vi "stim points to waveform.vi"(0 "stim point array":cluster{"X":u32, "Y":u32}[](array[cluster])=[{"X"=160, "Y"=192}, {"X"=107, "Y"=81}], 1 "stim power (%)":dbl(slide) scale=0.0..100.0, 2 "stim duration (in seconds)":dbl=5e-05 min=1e-05 max=0.002 step=1e-05 format="%#_6p", 3 "spot repetitions":dbl=1.0 min=1.0 step=1.0, 4 "group repetitions":dbl=1.0 min=1.0 step=1.0, 5 "pockels cell max power":dbl, 7 "stim interval (in seconds)":dbl=5e-05 min=5e-05 max=1.0 step=0.005 format="%#_6p", 9 "pre-stim settling time (in seconds)":dbl=5e-05 min=0.0 max=0.1 step=0.0001 format="%#_6p") -> (14 "x-y mirror data out":waveform(dbl)[](array[waveform]), 15 "pockels and piezo data out":waveform(dbl)[](array[waveform]), 16 "repetitions":dbl)   [LabVIEW 2012]
doc: "SciScan 1.2 160622"
panel:
  out "Waveform Graph 2":dbl[](graph)
  out "error out":errorcluster
  out "Waveform Graph":dbl[](graph)
  out "xyvoltagefor2frames":dbl[][][](array[numeric])
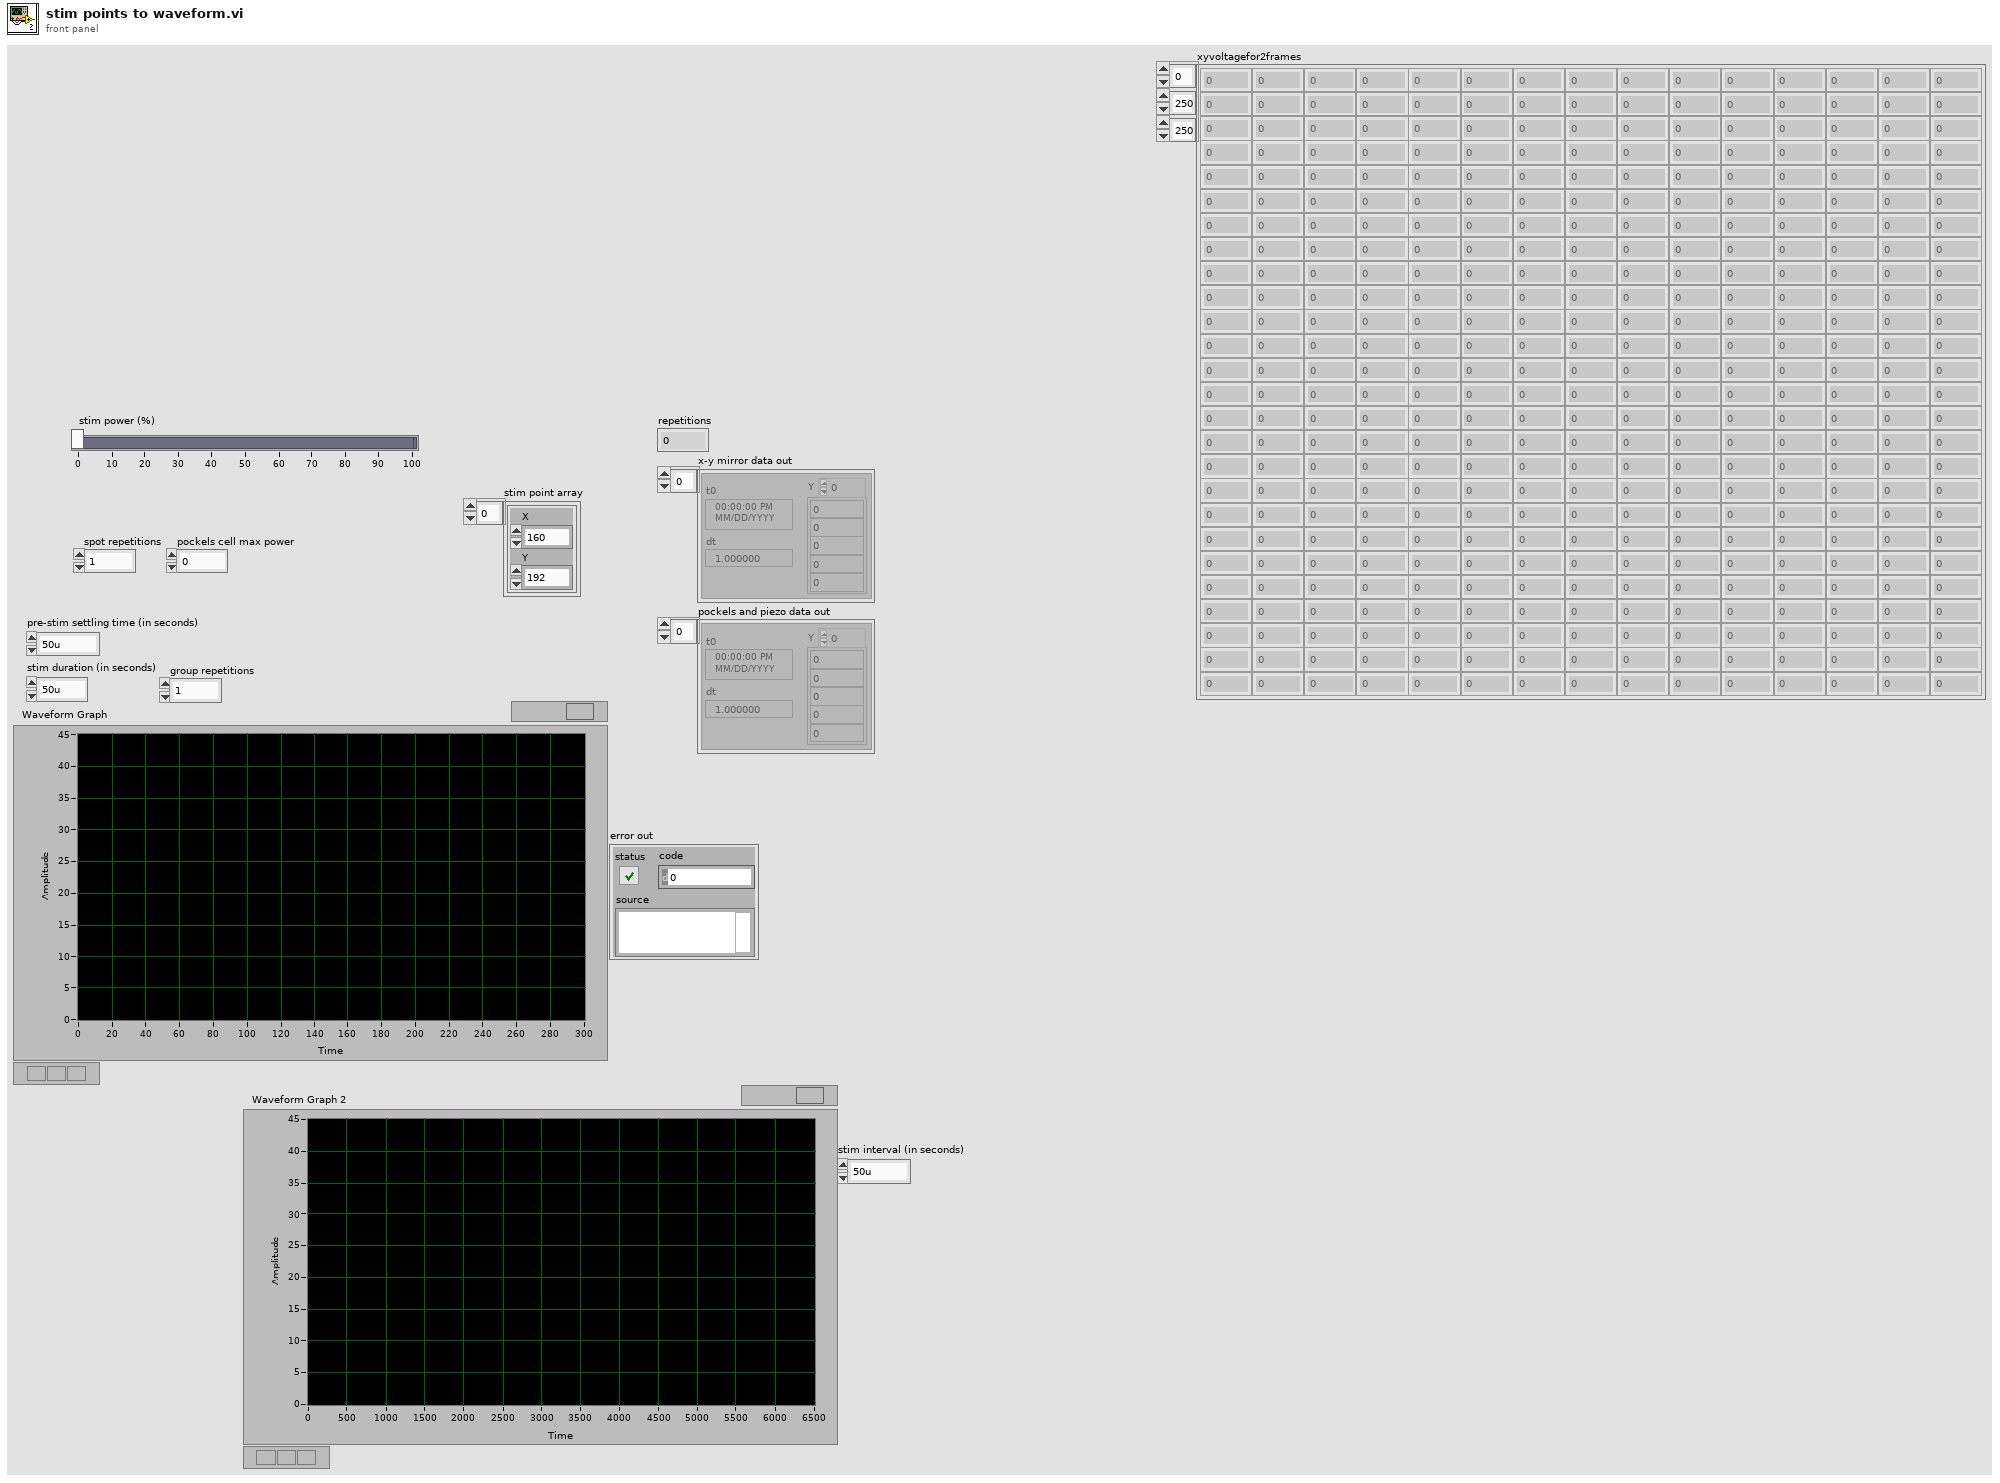
[diagram p1: front panel]
types:
  T1 = cluster{"xyvoltagefor2frames":dbl[][][], "x.pixels":dbl, "nomin.x.pixels":dbl, "y.pixels":dbl, "fill.fraction":dbl, "x.bidirectional":bool, "y.bidirectional":bool}
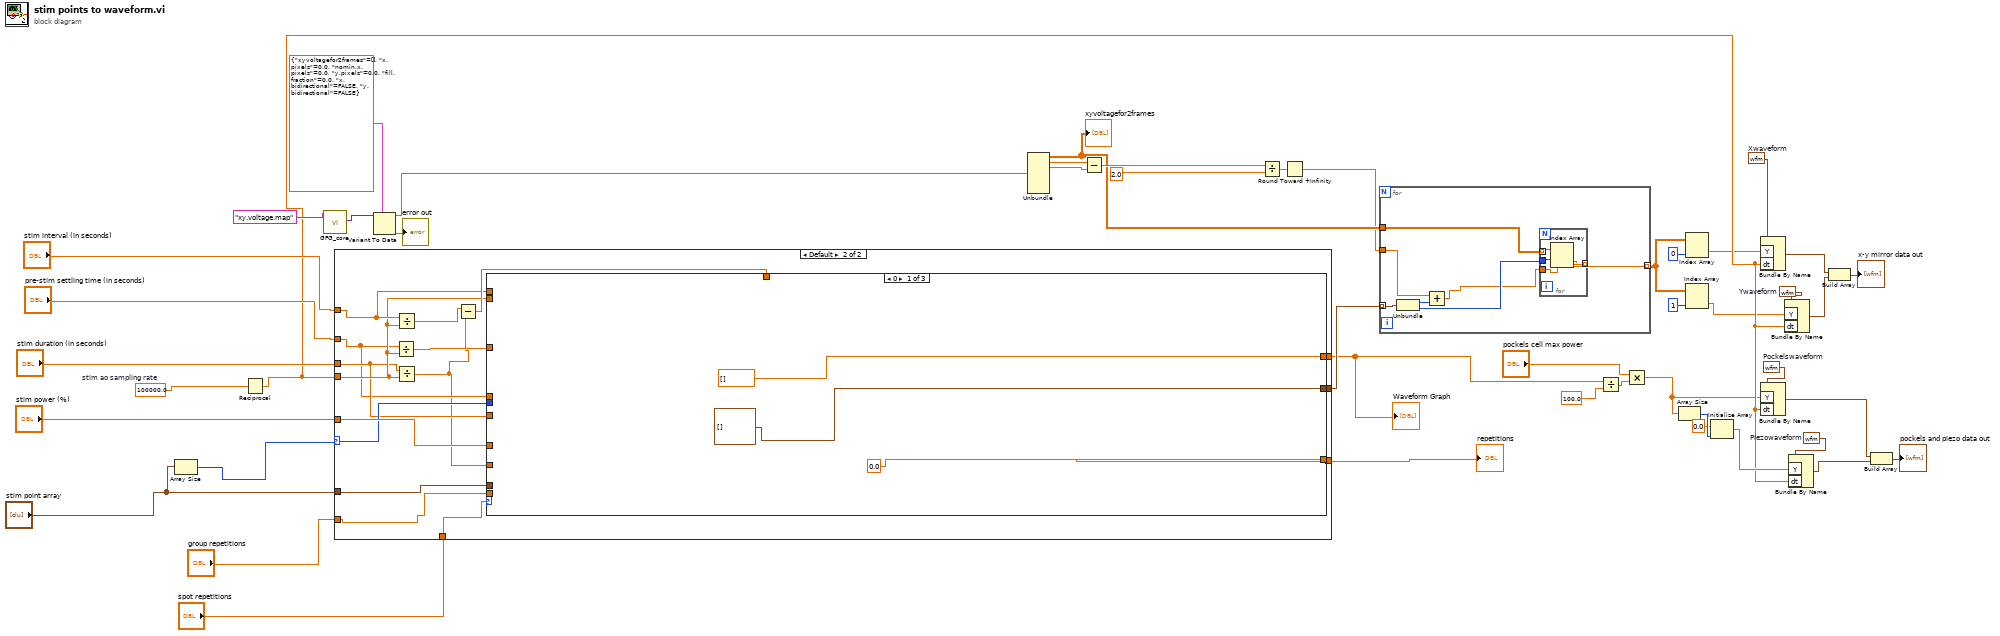
[diagram p0: block diagram]
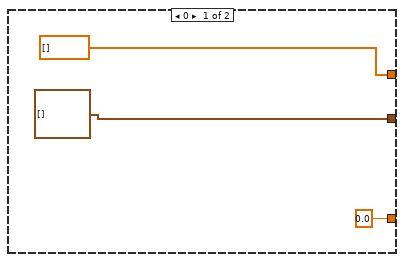
[diagram p2: hidden frame]
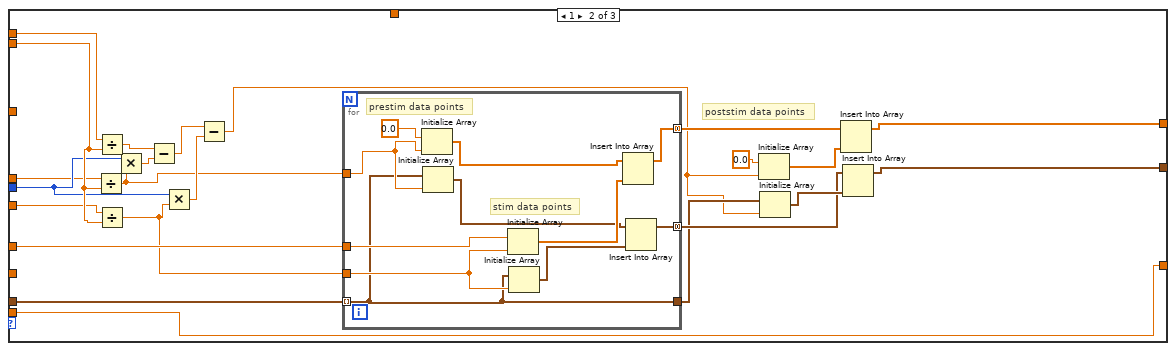
[diagram p3: hidden frame]
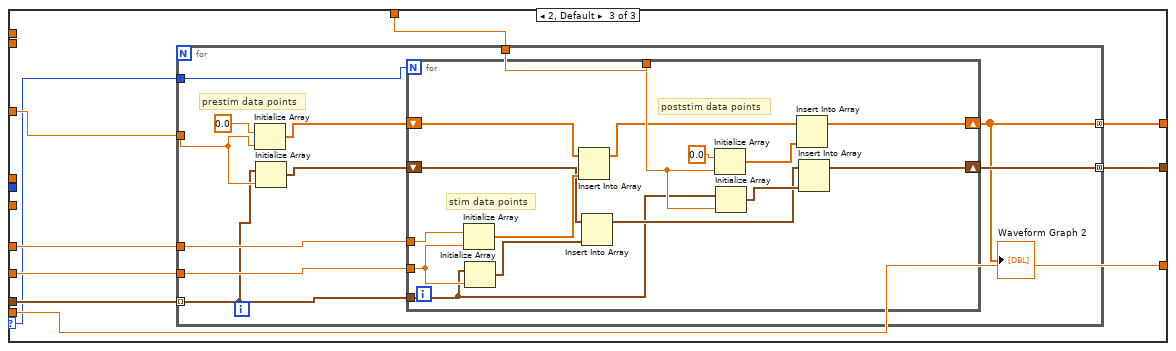
[diagram p4: hidden frame]
diagram:
  w10 = waveform(dbl) {"t0"=timestamp(0 s since 1904-01-01), "dt"=1.0, "Y"=[]}  # Piezowaveform
  w11 = waveform(dbl) {"t0"=timestamp(0 s since 1904-01-01), "dt"=1.0, "Y"=[]}  # Pockelswaveform
  w13 = waveform(dbl) {"t0"=timestamp(0 s since 1904-01-01), "dt"=1.0, "Y"=[]}  # Ywaveform
  w14 = waveform(dbl) {"t0"=timestamp(0 s since 1904-01-01), "dt"=1.0, "Y"=[]}  # Xwaveform
  w20 = 100000.0  # stim ao sampling rate
  n1 = Array Size(array="stim point array") -> (size(s)=w43:i32)
  n2 = Reciprocal(x=w20) -> (1/x=w16:dbl)
  n3 = call "GFG_core.vi"("Variable Name in"="xy.voltage.map") -> ("Variant Out"=w46:variant)  [unwired: 12 in, 6 out]
  n4 = case shown="Default" w43 {
    selector: w43 -> [_ w56]
    tunnel: "stim point array" -> [_ w61]
    tunnel: "stim interval (in seconds)" -> [_ w58]
    tunnel: "pre-stim settling time (in seconds)" -> [_ w54]
    tunnel: "stim power (%)" -> [_ w66]
    tunnel: w16 -> [_ w57]
    tunnel: "stim duration (in seconds)" -> [_ w55]
    tunnel: [dbl[] [] w64] -> w2
    tunnel: [cluster{"X":u32, "Y":u32}[] [] w63] -> w27
    tunnel: [0.0 ("group repetitions") w59] -> w37
    tunnel: "spot repetitions" -> [_ w62]
    tunnel: "group repetitions" -> [_ w60]
    frame 0 {
    }
    frame Default {
      n5 = Divide(x=w54, y=w57) -> (x/y=w53:dbl)
      n6 = Divide(x=w58, y=w57) -> (x/y=w51:dbl)
      n7 = Divide(x=w55, y=w57) -> (x/y=w52:dbl)
      n8 = Subtract(x=w51, y=w52) -> (x-y=w65:dbl)
      n9 = case shown="0" w62 {
        selector: w62 -> [_ _ w105]
        tunnel: w66 -> [_ w92 w112]
        tunnel: w53 -> [_ _ w111]
        tunnel: w52 -> [_ _ w110]
        tunnel: w65 -> [_ _ w109]
        tunnel: [dbl[] [] w91 w104] -> w64
        tunnel: [cluster{"X":u32, "Y":u32}[] [] w90 w108] -> w63
        tunnel: w61 -> [_ w89 w106]
        tunnel: w60 -> [_ w82 w107]
        tunnel: [0.0 ("group repetitions") w82 w107] -> w59
        tunnel: w58 -> [_ w77 _]
        tunnel: w57 -> [_ w76 _]
        tunnel: w56 -> [_ w75 _]
        tunnel: w55 -> [_ w74 _]
        tunnel: w54 -> [_ w70 _]
        frame 0 {
        }
        frame 1 {
          # "poststim data points"
          n10 = Divide(x=w70, y=w76) -> (x/y=w73:dbl)
          n11 = Divide(x=w77, y=w76) -> (x/y=w78:dbl)
          n12 = Divide(x=w74, y=w76) -> (x/y=w72:dbl)
          n13 = Multiply(x=w75, y=w73) -> (x*y=w81:dbl)
          n14 = Subtract(x=w78, y=w81) -> (x-y=w79:dbl)
          n15 = Multiply(x=w75, y=w72) -> (x*y=w80:dbl)
          n16 = Subtract(x=w79, y=w80) -> (x-y=w71:dbl)
          n17 = for {
            tunnel: w92 -> [w103]
            tunnel: w73 -> [w102]
            tunnel: w72 -> [w101]
            tunnel: w89 -> [w93] mode=indexing
            tunnel: [w97] -> w87 mode=concatenating
            tunnel: [w94] -> w84 mode=concatenating
            tunnel: [w93] -> w83
            # "prestim data points"
            # "stim data points"
            n18 = Initialize Array(0.0 ("stim power (%)"), w102) -> (w99:dbl[])
            n19 = Initialize Array(w93, w102) -> (w96:cluster{"X":u32, "Y":u32}[])
            n20 = Initialize Array(w103, w101) -> (w98:dbl[])
            n21 = Initialize Array(w93, w101) -> (w95:cluster{"X":u32, "Y":u32}[])
            n22 = Insert Into Array(array=w99, new element=w98) -> (w97:dbl[])  [unwired: 1 in]
            n23 = Insert Into Array(array=w96, new element=w95) -> (w94:cluster{"X":u32, "Y":u32}[])  [unwired: 1 in]
          }
          n24 = Initialize Array(0.0 ("stim power (%)"), w71) -> (w86:dbl[])
          n25 = Initialize Array(w83, w71) -> (w85:cluster{"X":u32, "Y":u32}[])
          n26 = Insert Into Array(array=w87, new element=w86) -> (w91:dbl[])  [unwired: 1 in]
          n27 = Insert Into Array(array=w84, new element=w85) -> (w90:cluster{"X":u32, "Y":u32}[])  [unwired: 1 in]
        }
        frame 2, Default {
          n28 = for {
            tunnel: w112 -> [w123]
            tunnel: w111 -> [w122]
            tunnel: w110 -> [w121]
            tunnel: w109 -> [w120]
            tunnel: [w113] -> w104 mode=concatenating
            tunnel: [w114] -> w108 mode=concatenating
            tunnel: w106 -> [w116] mode=indexing
            tunnel: w105 -> [w115]
            # "prestim data points"
            n29 = Initialize Array(0.0 ("stim power (%)"), w122) -> (w118:dbl[])
            n30 = Initialize Array(w116, w122) -> (w117:cluster{"X":u32, "Y":u32}[])
            n31 = for {
              N: w115 -> [_]
              tunnel: w123 -> [w138]
              tunnel: w121 -> [w137]
              tunnel: w120 -> [w136]
              tunnel: w116 -> [w130]
              shift-right: [w124] -> w113
              shift-left: w118 -> [w129]
              shift-right: [w125] -> w114
              shift-left: w117 -> [w127]
              # "stim data points"
              # "poststim data points"
              n32 = Initialize Array(w138, w137) -> (w128:dbl[])
              n33 = Initialize Array(w130, w137) -> (w126:cluster{"X":u32, "Y":u32}[])
              n34 = Insert Into Array(array=w129, new element=w128) -> (w134:dbl[])  [unwired: 1 in]
              n35 = Insert Into Array(array=w127, new element=w126) -> (w131:cluster{"X":u32, "Y":u32}[])  [unwired: 1 in]
              n36 = Initialize Array(0.0 ("stim power (%)"), w136) -> (w133:dbl[])
              n37 = Initialize Array(w130, w136) -> (w132:cluster{"X":u32, "Y":u32}[])
              n38 = Insert Into Array(array=w134, new element=w133) -> (w124:dbl[])  [unwired: 1 in]
              n39 = Insert Into Array(array=w131, new element=w132) -> (w125:cluster{"X":u32, "Y":u32}[])  [unwired: 1 in]
            }
            "Waveform Graph 2" <- w113
          }
        }
      }
    }
  }
  "repetitions" <- w37
  "Waveform Graph" <- w2
  n40 = Variant To Data(type=T1 {"xyvoltagefor2frames"=[], "x.pixels"=0.0, "nomin.x.pixels"=0.0, "y.pixels"=0.0, "fill.fraction"=0.0, "x.bidirectional"=FALSE, "y.bidirectional"=FALSE} ("output cluster"), Variant=w46) -> (data=w31:T1, error out=→"error out":errorcluster)  [unwired: 1 in]
  n41 = Unbundle(w31) -> ("xyvoltagefor2frames"=w30:dbl[][][], "x.pixels"=w28:dbl, "nomin.x.pixels"=w35:dbl)  [unwired: 4 out]
  "xyvoltagefor2frames" <- w30
  n42 = Subtract(x=w28, y=w35) -> (x-y=w32:dbl)
  n43 = Divide(x=w32, y=2.0) -> (x/y=w34:dbl)
  n44 = Round Toward +Infinity(x=w34) -> (ceil(x): smallest int >= x=w29:dbl)
  n45 = for {
    tunnel: w27 -> [w145] mode=indexing
    tunnel: [w143] -> w21 mode=indexing
    tunnel: w30 -> [w144]
    tunnel: w29 -> [w140]
    n46 = Unbundle(w145) -> ("X"=w141:u32, "Y"=w142:u32)
    n47 = Add(x=w140, y=w141) -> (x+y=w139:dbl)
    n48 = for {
      tunnel: w144 -> [w149] mode=indexing
      tunnel: w139 -> [w148]
      tunnel: w142 -> [w147]
      tunnel: [w146] -> w143 mode=indexing
      n49 = Index Array(array=w149, index (row)=w147, index (col)=w148) -> (element=w146:dbl)
    }
  }
  n50 = Divide(x=w2, y=100.0 ("x")) -> (x/y=w25:dbl[])
  n51 = Multiply(x="pockels cell max power", y=w25) -> (x*y=w3:dbl[])
  n52 = Array Size(array=w3) -> (size(s)=w19:i32)
  n53 = Index Array(array=w21, index (col)=0 ("disabled index (col)")) -> (element=w5:dbl[])  [unwired: 1 in]
  n54 = Index Array(array=w21, index (col)=1 ("disabled index (col)")) -> (element=w4:dbl[])  [unwired: 1 in]
  n55 = Initialize Array(0.0 ("element"), w19) -> (w17:dbl[])
  n56 = Bundle By Name(cluster=w14, "Y"=w5, "dt"=w16) -> (w15:waveform(dbl))
  n57 = Bundle By Name(cluster=w11, "Y"=w3, "dt"=w16) -> (w8:waveform(dbl))
  n58 = Bundle By Name(cluster=w13, "Y"=w4, "dt"=w16) -> (w12:waveform(dbl))
  n59 = Bundle By Name(cluster=w10, "Y"=w17, "dt"=w16) -> (w9:waveform(dbl))
  n60 = Build Array(w15, w12) -> (→"x-y mirror data out":waveform(dbl)[])
  n61 = Build Array(w8, w9) -> (→"pockels and piezo data out":waveform(dbl)[])
